vi "macro_Input_Modulus.vi"   [LabVIEW 2019, in "Trajectory_Library.lvlib"]
uses:
  Trajectory_Library.lvlib
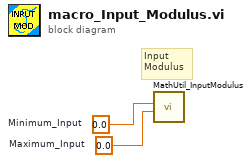
[diagram p0: block diagram]
diagram:
  w1 = 0.0  # Minimum_Input
  w2 = 0.0  # Maximum_Input
  # "Input\nModulus"
  n1 = call "MathUtil_InputModulus.vi"("Maximum_Input"=w2, "Minimum_Input"=w1) -> ()  [unwired: 9 in, 1 out]
